vi "piston toggle.vi"(9 "invert?":bool, 10 "refnum":string, 11 "intput":bool) -> ()   [LabVIEW 2016]
uses:
  <vilib>/Rock Robotics/WPI/Solenoid/WPI_SolenoidValue.ctl
  <vilib>/Rock Robotics/WPI/Solenoid/WPI_SolenoidSetEnum.vi
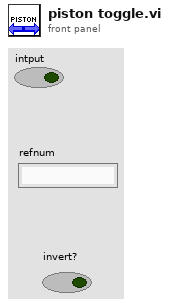
[diagram p1: front panel]
types:
  T1 = typedef "WPI_SolenoidDevRef.ctl" = cluster{"DevStatus":errorcluster, "Pneumatics Control Module":u8, "Forward Solenoid Channel":T2, "Reverse Solenoid Channel":T2}
  T2 = typedef "WPI_SolenoidChannel.ctl" = enum8{"Solenoid 0", "Solenoid 1", "Solenoid 2", "Solenoid 3", "Solenoid 4", "Solenoid 5", "Solenoid 6", "Solenoid 7", "Invalid"}
  T3 = typedef "WPI_SolenoidValue.ctl" = enum16{"Off", "On", "Forward", "Reverse"}
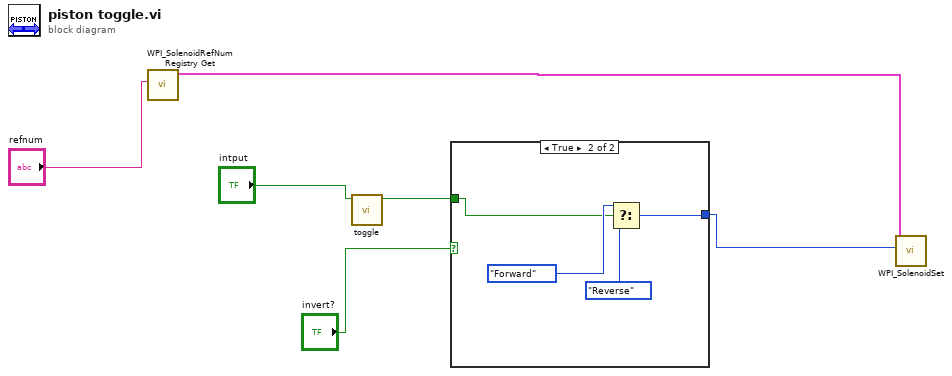
[diagram p0: block diagram]
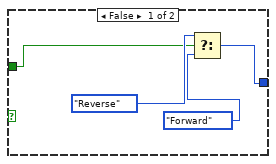
[diagram p2: hidden frame]
diagram:
  n1 = call <vilib>:"WPI_SolenoidRefNum Registry Get.vi"("refnum name"="refnum") -> ("SolenoidDevRef"=w5:T1)  [unwired: 9 in, 1 out]
  n2 = call "toggle.vi"("Boolean"="intput") -> ("Boolean 2"=w2:bool)  [unwired: 10 in]
  n3 = case shown="True" "invert?" {
    tunnel: [w9 w12] -> w1
    tunnel: w2 -> [w7 w11]
    frame False {
      n4 = Select(t=WPI_SolenoidValue."Reverse" ("Value"), s=w7, f=WPI_SolenoidValue."Forward" ("Value")) -> (s? t:f=w9:T3)
    }
    frame True {
      n5 = Select(t=WPI_SolenoidValue."Forward" ("Value"), s=w11, f=WPI_SolenoidValue."Reverse" ("Value")) -> (s? t:f=w12:T3)
    }
  }
  n6 = call-poly <vilib>:"WPI_SolenoidSet.vi"("Value"=w1, "SolenoidDevRef"=w5) -> ()  [unwired: 8 in, 2 out]
